vi "SplitStringToArray.vi"(8 "offset (0)":i32, 10 "search string/char (-)":string, 11 "String in":string) -> (3 "Split(s)":string[](array[string]))   [LabVIEW 2017]
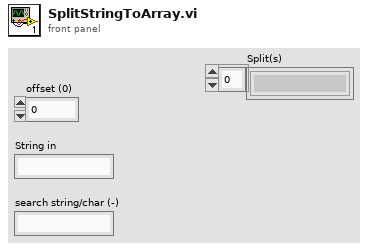
[diagram p1: front panel]
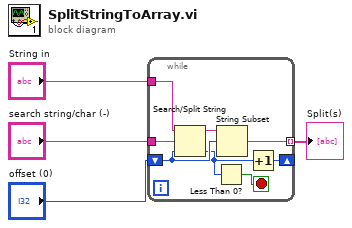
[diagram p0: block diagram]
diagram:
  n1 = while {
    tunnel: "search string/char (-)" -> [w12]
    tunnel: "String in" -> [w11]
    tunnel: [w8] -> w2 mode=indexing
    shift-right: [w7] -> _
    shift-left: "offset (0)" -> [w10]
    stop <- w6 stop-if-true
    n2 = Search/Split String(string=w11, search string/char (-)=w12, offset (0)=w10) -> (substring before match=w9:string, offset of match=w5:i32)  [unwired: 1 out]
    n3 = Less Than 0?(x=w5) -> (x < 0?=w6:bool)
    n4 = String Subset(string=w9, offset (0)=w10) -> (substring=w8:string)  [unwired: 1 in]
    n5 = Increment(x=w5) -> (x+1=w7:i32)
  }
  "Split(s)" <- w2
